vi "Stop Core.vi"(10 "最终错误代码":i32, 11 "Task A输入":refnum<class "Task A.lvclass">) -> (3 "Task A输出":refnum<class "Task A.lvclass">)   [LabVIEW 2013, in "Task A操作者.lvlib" / "Task A.lvclass"]
uses:
  Task A.lvclass
  <vilib>/ActorFramework/Time-Delayed Send Message/Time-Delay Override Options.ctl
  <vilib>/ActorFramework/Actor/Actor.lvclass
  Task A.lvclass/Task A.ctl
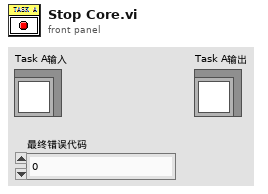
[diagram p1: front panel]
types:
  T1 = typedef "Time-Delay Override Options.ctl" = enum16{"Send next copy now", "Skip next scheduled copy", "Send next copy now and stop all further copies", "Stop all further copies"}
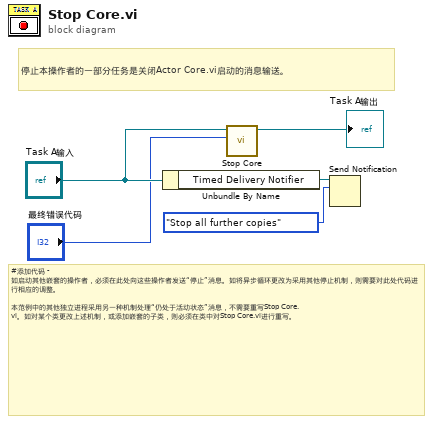
[diagram p0: block diagram]
diagram:
  # "#添加代码 - 如启动其他嵌套的操作者，必须在此处向这些操作者发送“停止”消息。如将异步循环更改为采用其他停止机制，则需要对此处代码进行相应的调整。\n\n本范例中的其他独立进程采用另一种机制处理“仍处于活动状态”消息，不需要重写Stop Core.vi。如对某个类更改上述机制，或添加嵌套的子类，则必须在类中对Stop Core.vi进行重写。"
  # "停止本操作者的一部分任务是关闭Actor Core.vi启动的消息输送。"
  n1 = Unbundle By Name("Task A输入") -> ("Timed Delivery Notifier"=w3:refnum<notifier>)
  n2 = call-parent "Stop Core.vi"("final error code"="最终错误代码", "Actor in"="Task A输入") -> ("Actor out"=→"Task A输出":refnum<class "Task A.lvclass">)  [unwired: 9 in]
  n3 = Send Notification(notification=Time-Delay_Override_Options."Stop all further copies", notifier=w3) -> ()  [unwired: 1 in, 2 out]
